vi "Config - Search.vi"(8 "error in (no error)":errorcluster, 10 "Account Number":i32, 11 "Config Data Array":T1[](array[typedef])) -> (0 "error out":errorcluster, 2 "Not Found":bool, 3 "Config Data":T1)   [LabVIEW 2017]
doc: "Provides search mechanism based upon an Account Number in the configuration data records."
uses:
  Controls/Config Data.ctl
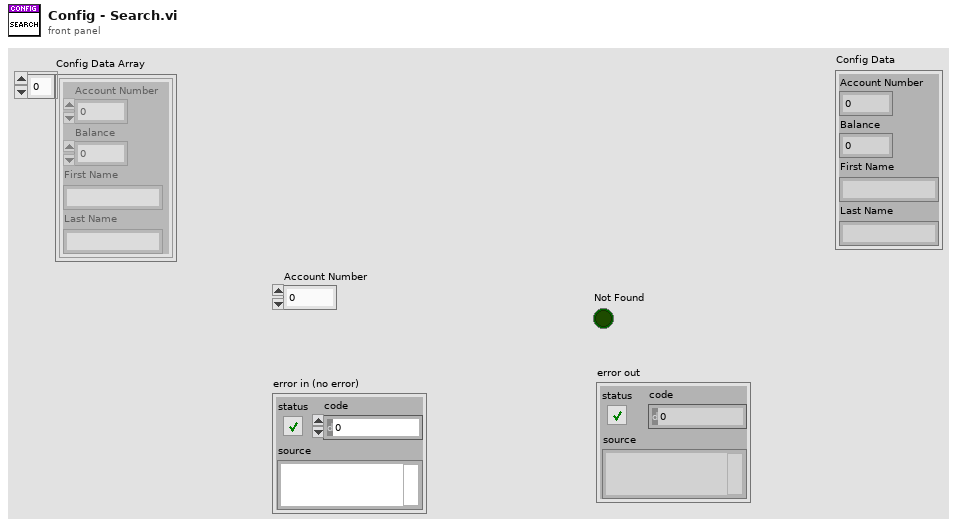
[diagram p1: front panel]
types:
  T1 = typedef "Config Data.ctl" = cluster{"Account Number":i32, "Balance":dbl, "First Name":string, "Last Name":string}
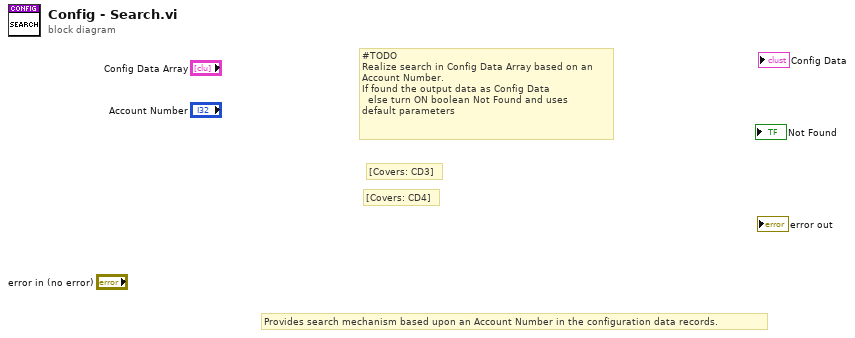
[diagram p0: block diagram]
diagram:
  # "[Covers: CD4]"
  # "[Covers: CD3]"
  # "Provides search mechanism based upon an Account Number in the configuration data records."
  # "#TODO\nRealize search in Config Data Array based on an\nAccount Number.\nIf found the output data as Config Data\n  else turn ON boolean Not Found and uses \ndefault parameters"
